vi "Wait Log.vi"(8 "error in":errorcluster, 11 "Log Data":string) -> (0 "error out":errorcluster)   [LabVIEW 2023, in "HardwareAbstractionLayer_LVOOP.lvlib" / "Wait Monitor.lvclass"]
uses:
  Wait Monitor.lvclass
  Database/Database.lvclass
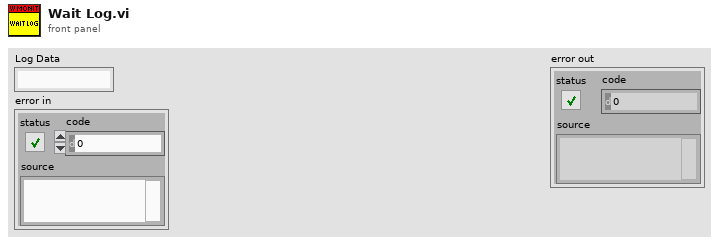
[diagram p1: front panel]
types:
  T1 = enum16{"open", "replace", "create", "open or create", "replace or create", "replace or create with confirmation"}
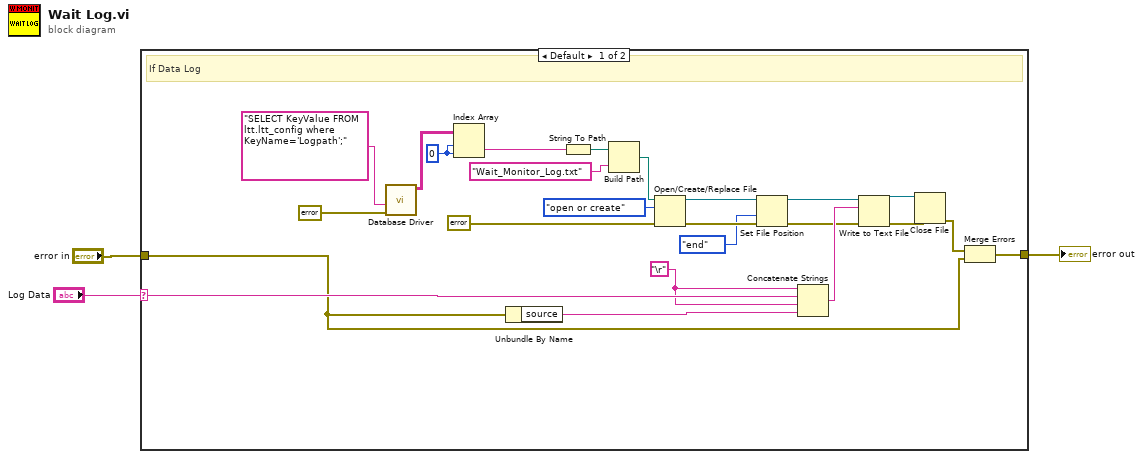
[diagram p0: block diagram]
diagram:
  n1 = case shown="Default" "Log Data" {
    selector: "Log Data" -> [w27 _]
    tunnel: [w10 w28] -> w2
    tunnel: "error in" -> [w4 w28]
    frame Default {
      w15 = "\r"
      w20 = 0 ("disabled index (col)")
      # "If Data Log"
      n2 = call "Database Driver.vi"("error in"=errorcluster {"status"=FALSE, "code"=0, "source"=""} ("error in (no error)"), "SQL query"="SELECT KeyValue FROM ltt.ltt_config where KeyName='Logpath';") -> ("data"=w11:string[][])  [unwired: 6 in, 3 out]
      n3 = Index Array(array=w11, index (row)=w20, index (col)=w20) -> (element=w19:string)
      n4 = Unbundle By Name(w4) -> ("source"=w14:string)
      n5 = String To Path(string=w19) -> (path=w18:path)
      n6 = Build Path(base path=w18, name or relative path="Wait_Monitor_Log.txt") -> (appended path=w22:path)
      n7 = Open/Create/Replace File(file path (use dialog)=w22, error in=errorcluster {"status"=FALSE, "code"=0, "source"=""}, operation (0:open)=T1."open or create") -> (refnum out=w9:refnum<file>, error out=w8:errorcluster)  [unwired: 3 in, 1 out]
      n8 = Set File Position(refnum=w9, from (0:start)=enum16{"start", "end", "current"}."end", error in=w8) -> (refnum out=w6:refnum<file>, error out=w7:errorcluster)  [unwired: 1 in]
      n9 = Concatenate Strings(w15, w27, w15, w14) -> (w16:string)
      n10 = Write to Text File(file (use dialog)=w6, text=w16, error in=w7) -> (refnum out=w26:refnum<file>, error out=w25:errorcluster)  [unwired: 1 in, 1 out]
      n11 = Close File(refnum=w26, error in=w25) -> (error out=w21:errorcluster)  [unwired: 1 out]
      n12 = Merge Errors(w21, w4) -> (w10:errorcluster)
    }
    frame "" {
      # "Emety Not Log"
    }
  }
  "error out" <- w2
